vi "Farming Robot V1.vi"() -> ()   [LabVIEW 2021]
uses:
  <vilib>/myRIO/Express VI/Onboard Devices/LED/LED Express VI.xnode
  <vilib>/myRIO/Instrument Drivers/Onboard IO/DIO/vis/Write.vi
  <vilib>/myRIO/Instrument Drivers/Onboard IO/DIO/DIO.lvlib
  <vilib>/myRIO/Common/Instrument Driver Framework/myRIO v1.0/DIO/typedefs/DIO Channels Enum.ctl
  <vilib>/myRIO/Common/Instrument Driver Framework/myRIO v1.0/DIO/typedefs/DIO Channels List.ctl
  <vilib>/myRIO/Common/Instrument Driver Framework/Utilities/typedefs/Generic FPGA Reference.ctl
  <vilib>/myRIO/Common/Instrument Driver Framework/Utilities/typedefs/myRIO v1.0 Reference.ctl
  <vilib>/myRIO/Common/Instrument Driver Framework/Utilities/typedefs/Hardware Version Enum.ctl
  <vilib>/myRIO/Common/Instrument Driver Framework/Utilities/typedefs/myRIO Generic Hardware Reference.ctl
  <vilib>/myRIO/Instrument Drivers/Onboard IO/DIO/typedefs/DIO Reference.ctl
  <vilib>/myRIO/Instrument Drivers/Onboard IO/DIO/vis/myRIO DIO Open.xnode
  <vilib>/myRIO/Common/Instrument Driver Framework/Utilities/vis/Is FPGA Ref Available.vi
  <vilib>/myRIO/Common/Instrument Driver Framework/myRIO v1.0/DIO/vis/myRIO v1.1 Open DIO.vi
  <vilib>/userDefined/High Color/nirio_resource_hc.ctl
  <vilib>/myRIO/Express VI/Onboard IO/DO/DO Express VI.xnode
  <vilib>/myRIO/Express VI/Onboard IO/PWM/PWM Express VI.xnode
  <vilib>/myRIO/Instrument Drivers/Onboard IO/PWM/vis/Set Duty Cycle and Frequency.vi
  <vilib>/myRIO/Instrument Drivers/Onboard IO/PWM/PWM.lvlib
  <vilib>/myRIO/Instrument Drivers/Onboard IO/PWM/typedefs/PWM Configuration.ctl
  <vilib>/myRIO/Common/Instrument Driver Framework/myRIO v1.0/PWM/typedefs/PWM Channels Enum.ctl
  <vilib>/myRIO/Instrument Drivers/Onboard IO/PWM/typedefs/PWM Reference.ctl
  <vilib>/myRIO/Instrument Drivers/Onboard IO/PWM/vis/myRIO PWM Open.xnode
  <vilib>/myRIO/Common/Instrument Driver Framework/myRIO v1.0/PWM/vis/myRIO v1.1 Open PWM.vi
  <vilib>/Analysis/NI_AALPro.lvlib
  <vilib>/myRIO/Express VI/Onboard Devices/Accelerometer/Accelerometer Express VI.xnode
  <vilib>/myRIO/Instrument Drivers/Onboard Devices/Accelerometer/vis/Read.vi
  <vilib>/myRIO/Instrument Drivers/Onboard Devices/Accelerometer/Accelerometer.lvlib
  <vilib>/myRIO/Common/Instrument Driver Framework/myRIO v1.0/Accelerometer/typedefs/Accelerometer Channels Enum.ctl
  <vilib>/myRIO/Common/Instrument Driver Framework/myRIO v1.0/Accelerometer/typedefs/Accelerometer Channels List.ctl
  <vilib>/myRIO/Instrument Drivers/Onboard Devices/Accelerometer/typedefs/Accelerometer Reference.ctl
  <vilib>/myRIO/Instrument Drivers/Onboard Devices/Accelerometer/vis/myRIO Accelerometer Open.xnode
  <vilib>/myRIO/Common/Instrument Driver Framework/myRIO v1.0/Accelerometer/vis/myRIO v1.1 Open Accelerometer.vi
panel:
  in  "servo 1":dbl(slide) scale=0.0..180.0
  out "pulse width 1":dbl
  out "Angle 1":dbl
  in  "Duty Cycle":dbl(slide)=0.5 scale=0.0..1.0
  in  "Input 4":bool
  in  "Input 3":bool
  in  "Input 2":bool
  in  "Input 1":bool
  in  "Start Farming":bool
  out "Watering":bool
  out "Seeding\nUp":bool
  out "Seeding\nDown":bool
  out "Switching\nMode":bool
  out "Drill Up":bool
  out "Drill Down":bool
  out "Intialize":bool
  out "Message":string
  in  "stop":bool
  out "States":T1(ring)
  # "Motors"
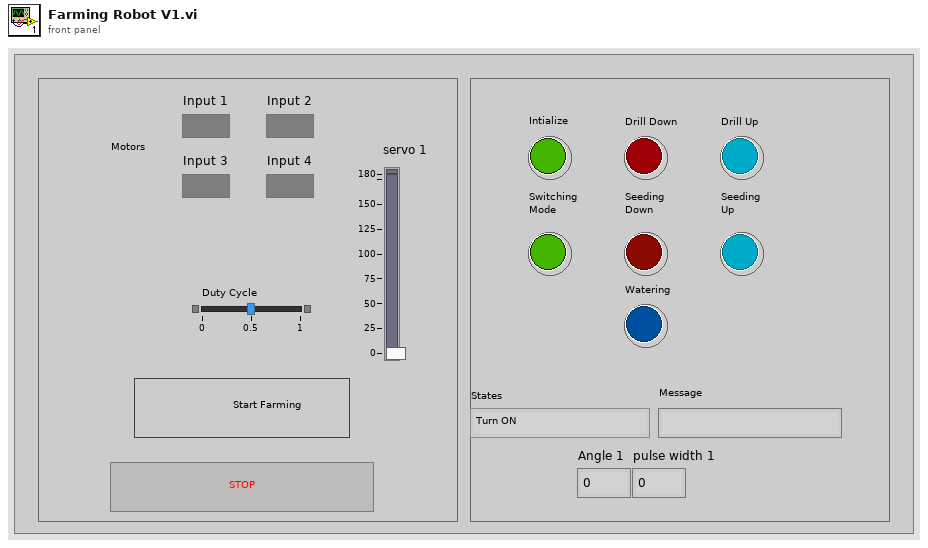
[diagram p1: front panel]
types:
  T1 = enum16{"Turn ON", "IDLE", "Start Farming", "Drive", "Seeding", "Watering", "Filling", "Fell off", "Stop", "Drill"}
  T2 = enum16{"Turn ON", "IDLE", "Start Farming", "Drive", "Seeding", "Watering", "Filling", "Fell off", "Stop"}
  T3 = typedef "DIO.lvlib/DIO Reference.ctl" = cluster{"myRIO Reference":T4, "DIO Channels List":T8}
  T4 = typedef "myRIO Generic Hardware Reference.ctl" = cluster{"myRIO Model":T5, "myRIO Hardware Reference":T6}
  T5 = typedef "Hardware Version Enum.ctl" = enum16{"Unknown", "myRIO-1900", "myRIO-1950", "roboRIO", "NI ELVIS RIO CM", "ELVIS III"}
  T6 = typedef "myRIO v1.0 Reference.ctl" = cluster{"Generic FPGA Reference":T7, "Allow multiple opens":bool}
  T7 = typedef "Generic FPGA Reference.ctl" = refnum<k20>
  T8 = typedef "DIO Channels List.ctl" = T9[]
  T9 = typedef "DIO Channels Enum.ctl" = enum16{"Not Connected", "C/DIO0", "C/DIO1", "C/DIO2", "C/DIO3", "C/DIO4", "C/DIO5", "C/DIO6", "C/DIO7", "A/DIO0", "A/DIO1", "A/DIO2", "A/DIO3", "A/DIO4", "A/DIO5", "A/DIO6", "A/DIO7", "A/DIO8", "A/DIO9", "A/DIO10", "A/DIO11", "A/DIO12", "A/DIO13", "A/DIO14", "A/DIO15", "A/DIO16", "A/DIO17", "A/DIO18", "A/DIO19", "B/DIO0", "B/DIO1", "B/DIO2", "B/DIO3", "B/DIO4", "B/DIO5", "B/DIO6", "B/DIO7", "B/DIO8", "B/DIO9", "B/DIO10", "B/DIO11", "B/DIO12", "B/DIO13", "B/DIO14", "B/DIO15", "B/DIO16", "B/DIO17", "B/DIO18", "B/DIO19", "LED0", "LED1", "LED2", "LED3", "Button0", "DIO/DIO0", "DIO/DIO1", "DIO/DIO2", "DIO/DIO3", "DIO/DIO4", "DIO/DIO5", "DIO/DIO6", "DIO/DIO7", "DIO/DIO8", "DIO/DIO9", "SPI/CS0", "SPI/CS1", "SPI/CS2", "SPI/CS3", "LED RADIO (Green)", "LED RADIO (Red)", "LED COMM (Green)", "LED COMM (Red)", "LED MODE (Green)", "LED MODE (Red)"}
  T10 = typedef "nirio_resource_hc.ctl" = tag
  T11 = typedef "Accelerometer.lvlib/Accelerometer Reference.ctl" = cluster{"myRIO Reference":T4, "Accelerometer Channels List":T12, "LSB Weight":dbl}
  T12 = typedef "Accelerometer Channels List.ctl" = T13[]
  T13 = typedef "Accelerometer Channels Enum.ctl" = enum16{"Not Connected", "X-Axis", "Y-Axis", "Z-Axis"}
  T14 = typedef "PWM.lvlib/PWM Reference.ctl" = cluster{"myRIO Reference":T4, "PWM Channels Enum":T15, "PWM Configuration":T16}
  T15 = typedef "PWM Channels Enum.ctl" = enum16{"Not Connected", "C/PWM0", "C/PWM1", "A/PWM0", "A/PWM1", "A/PWM2", "A/PWM3", "A/PWM4", "A/PWM5", "A/PWM6", "A/PWM7", "A/PWM8", "A/PWM9", "A/PWM10", "A/PWM11", "A/PWM12", "A/PWM13", "A/PWM14", "A/PWM15", "A/PWM16", "A/PWM17", "A/PWM18", "A/PWM19", "B/PWM0", "B/PWM1", "B/PWM2", "B/PWM3", "B/PWM4", "B/PWM5", "B/PWM6", "B/PWM7", "B/PWM8", "B/PWM9", "B/PWM10", "B/PWM11", "B/PWM12", "B/PWM13", "B/PWM14", "B/PWM15", "B/PWM16", "B/PWM17", "B/PWM18", "B/PWM19", "PWM/PWM0", "PWM/PWM1", "PWM/PWM2", "PWM/PWM3", "PWM/PWM4", "PWM/PWM5", "PWM/PWM6", "PWM/PWM7", "PWM/PWM8", "PWM/PWM9"}
  T16 = typedef "PWM.lvlib/PWM Configuration.ctl" = cluster{"Frequency":dbl, "Duty Cycle":dbl}
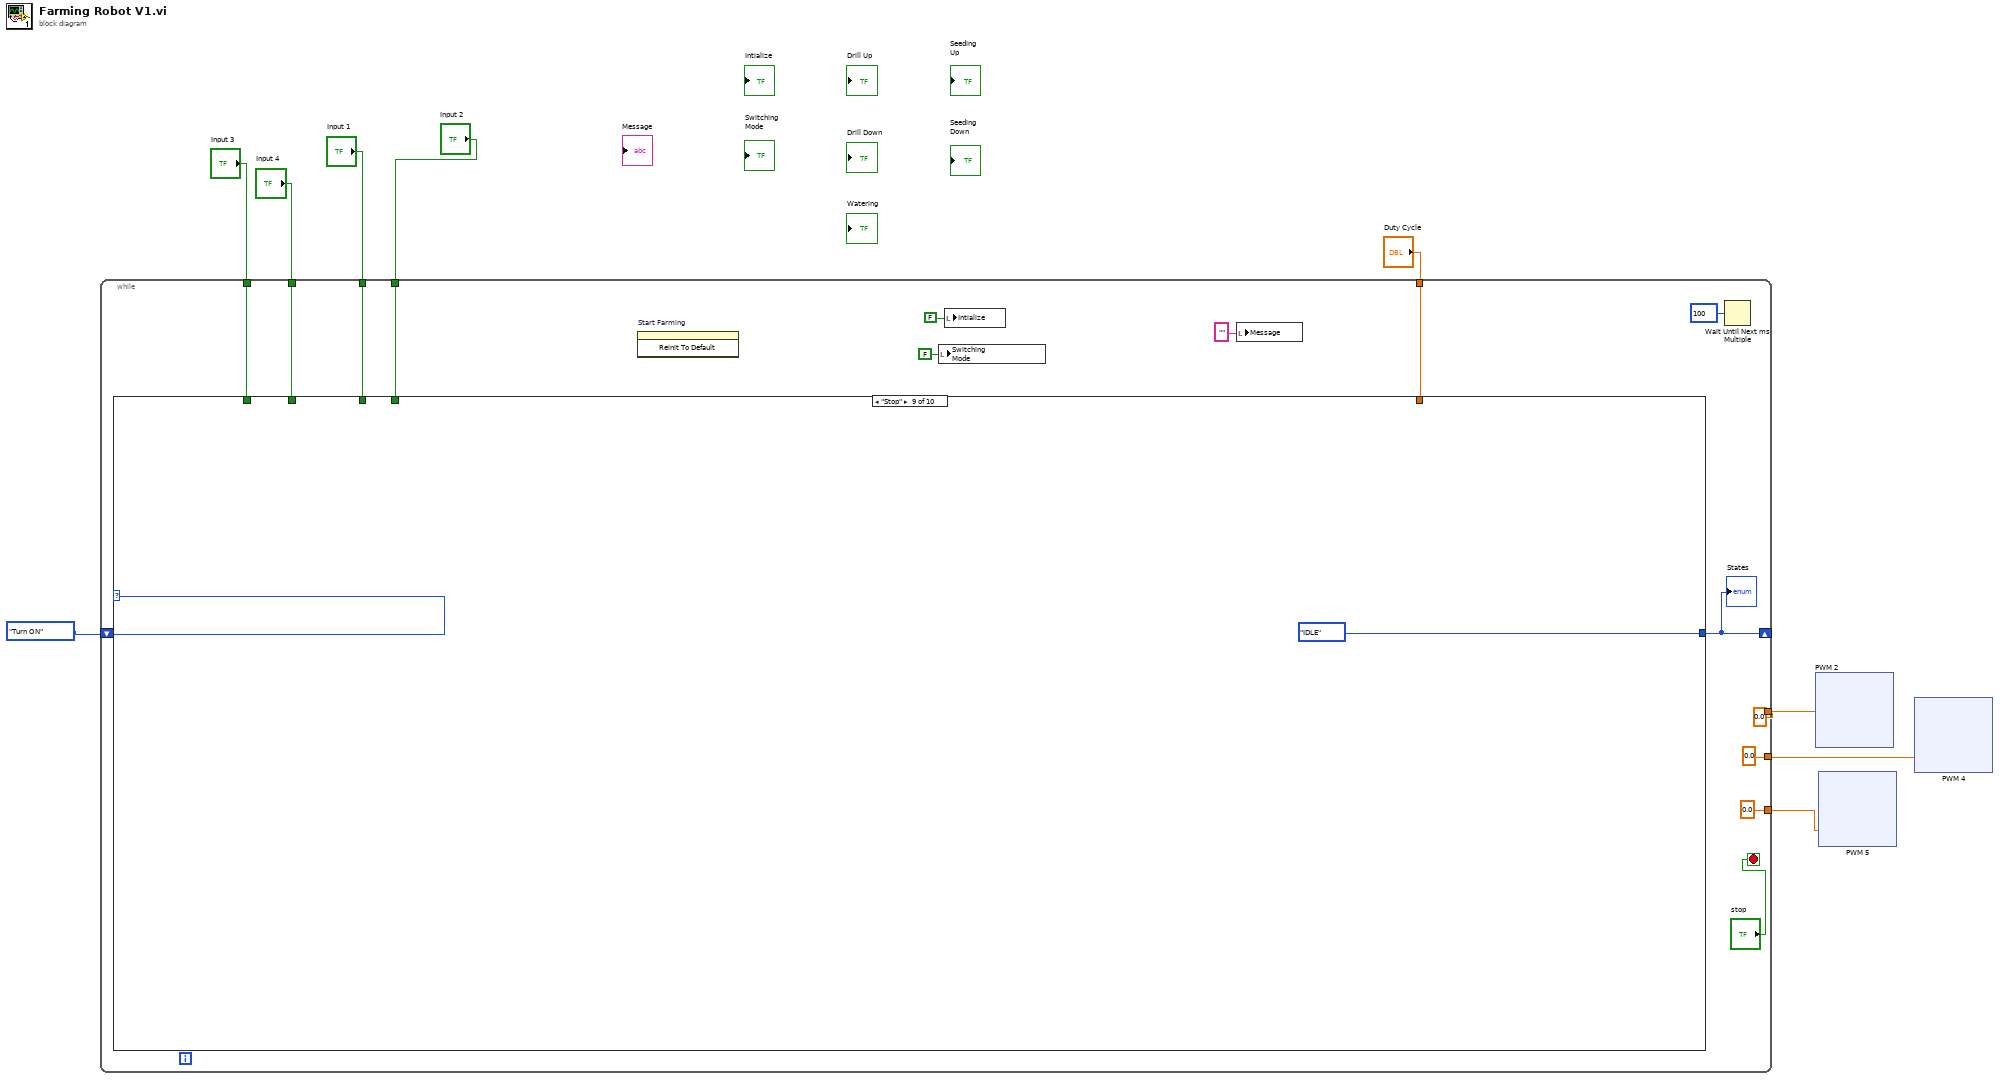
[diagram p0: block diagram]
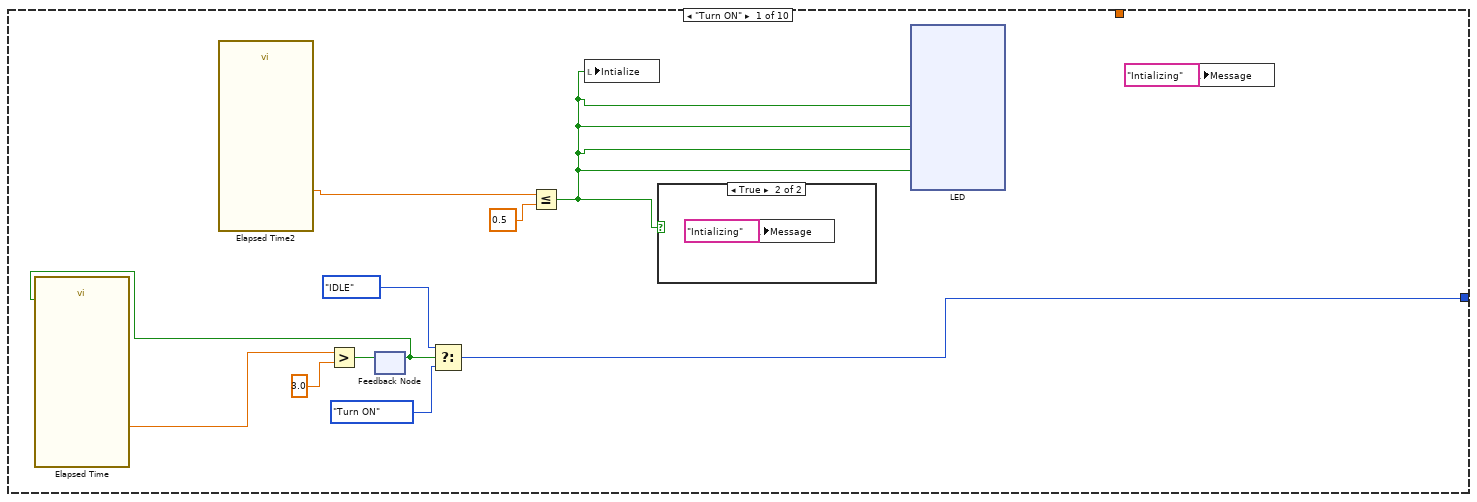
[diagram p2: hidden frame]
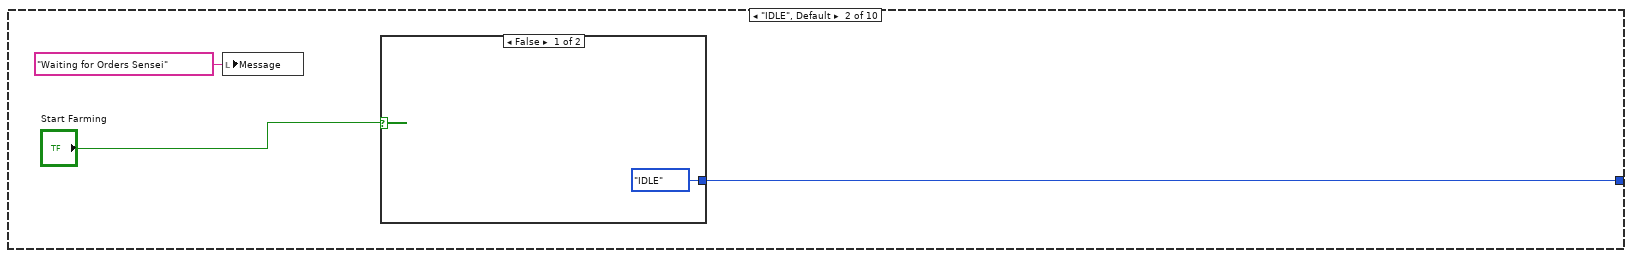
[diagram p4: hidden frame]
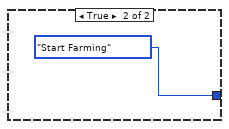
[diagram p5: hidden frame]
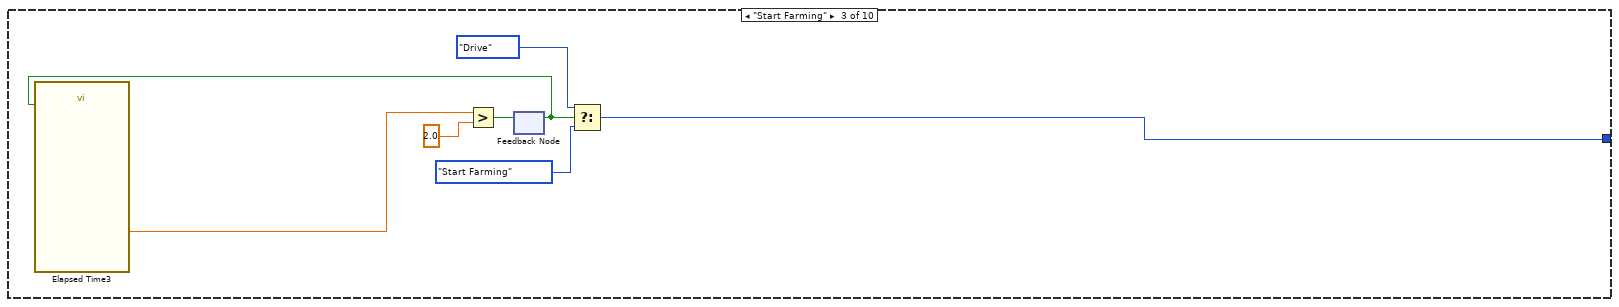
[diagram p6: hidden frame]
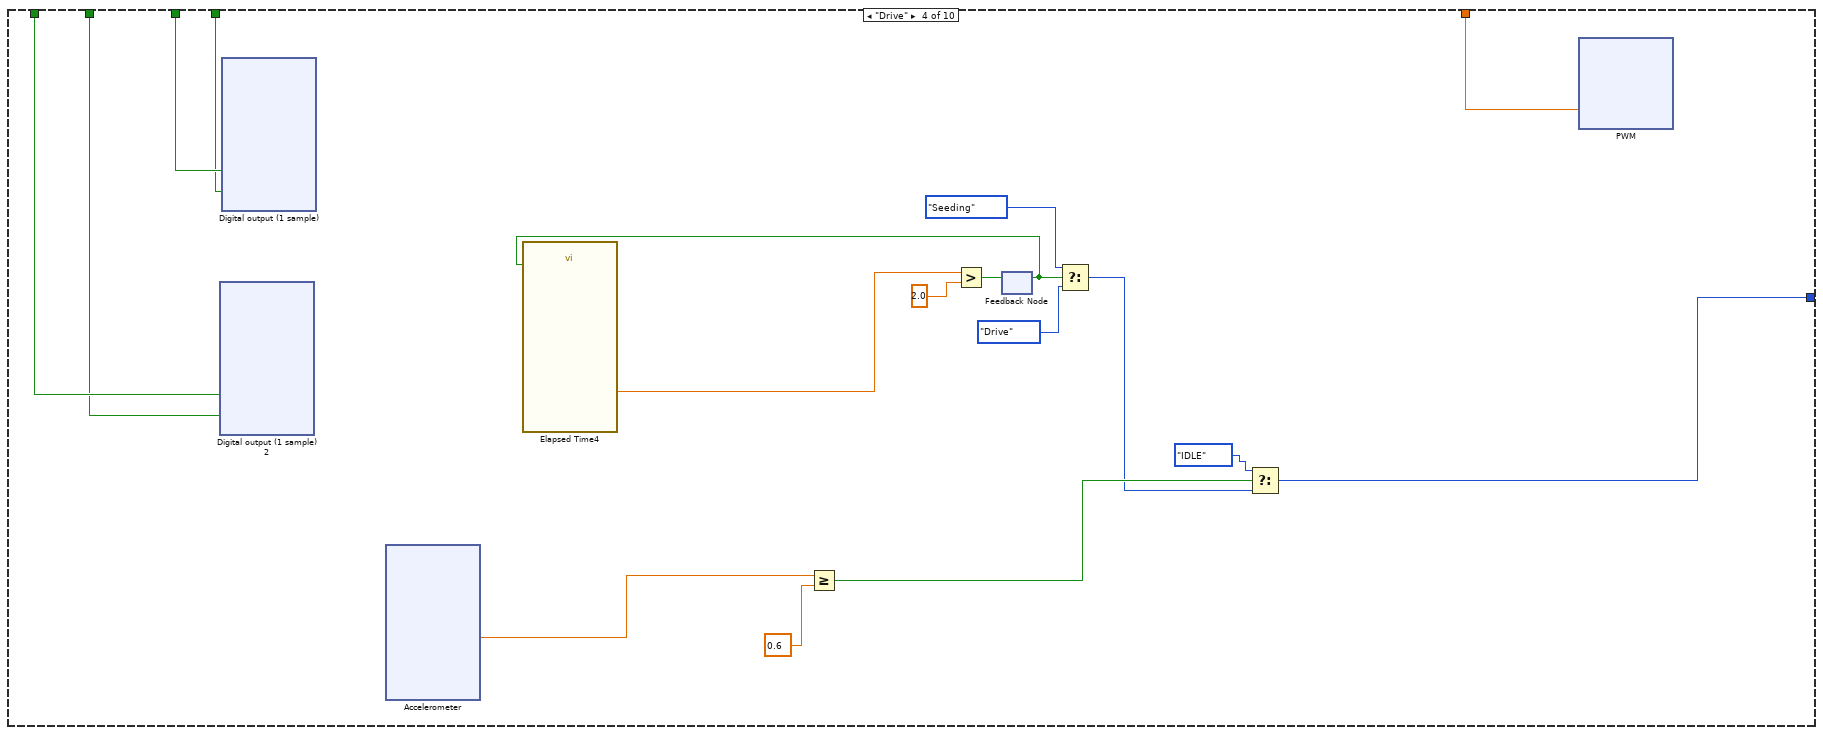
[diagram p7: hidden frame]
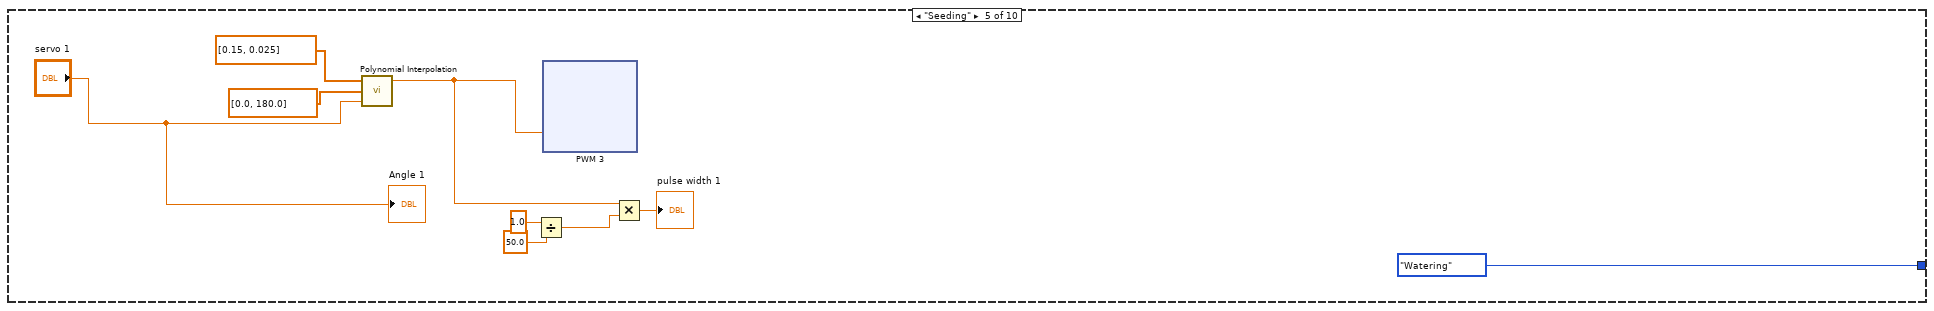
[diagram p8: hidden frame]
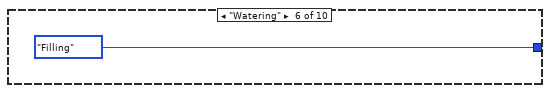
[diagram p9: hidden frame]
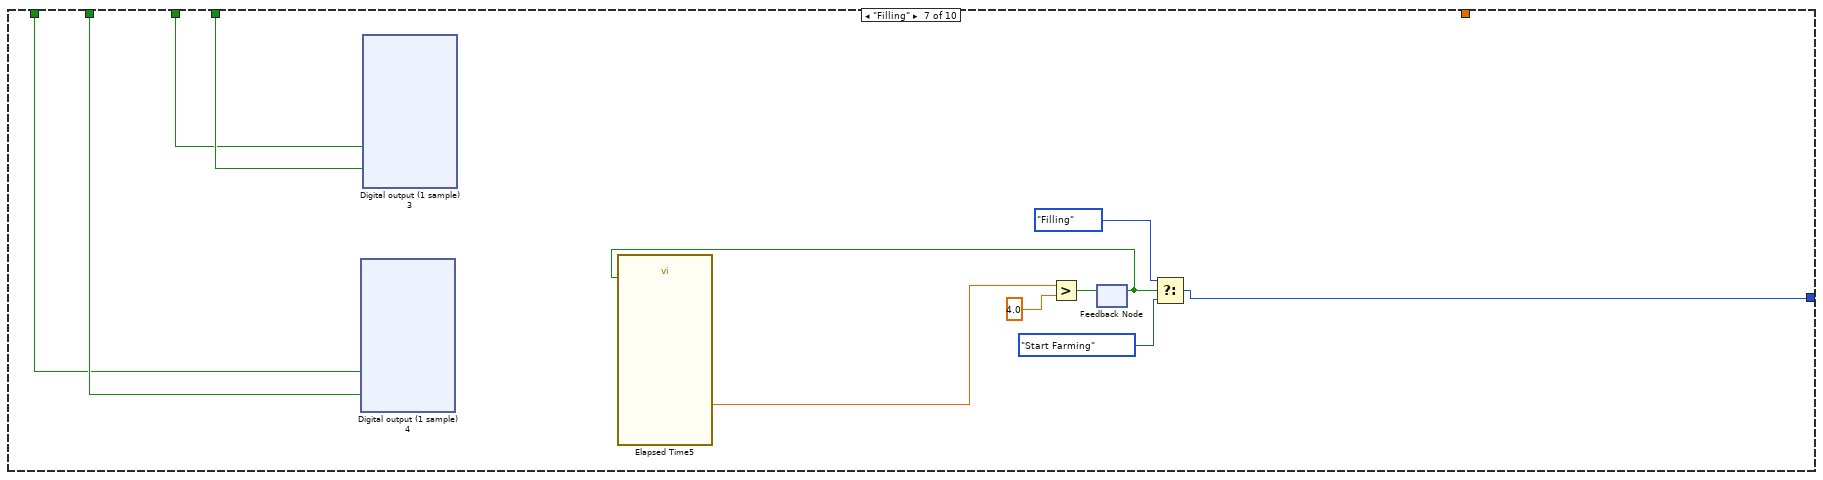
[diagram p10: hidden frame]
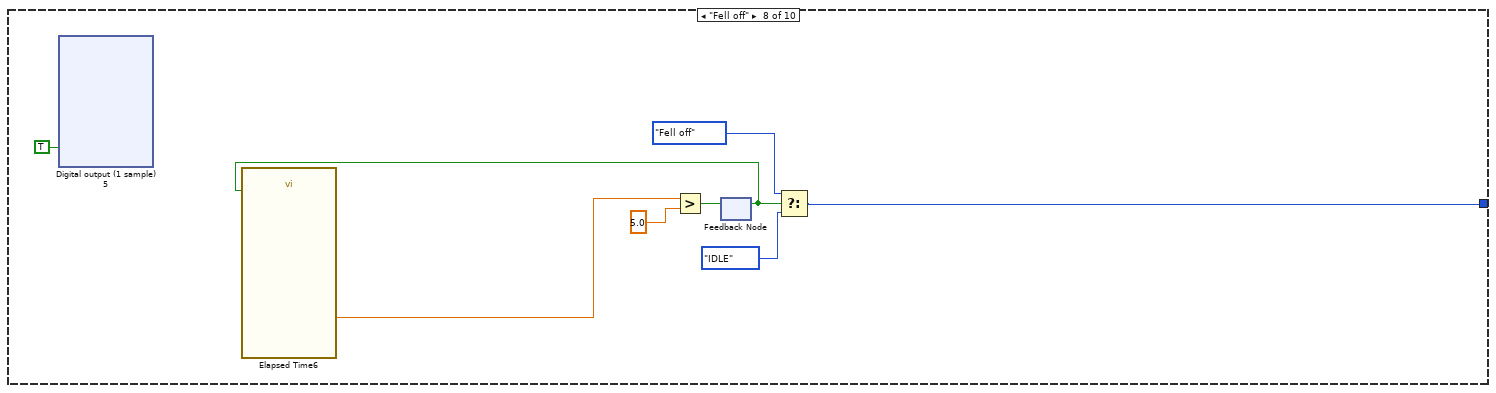
[diagram p11: hidden frame]
diagram:
  n1 = while {
    shift-right: [w22] -> _
    shift-left: T1."Turn ON" ("States") -> [w24]
    tunnel: [0.0 ("Duty Cycle")] -> w9
    tunnel: "Input 1" -> [w16]
    tunnel: "Input 2" -> [w15]
    tunnel: "Input 3" -> [w14]
    tunnel: "Input 4" -> [w13]
    tunnel: [0.0 ("Duty Cycle")] -> w4
    tunnel: [0.0 ("Duty Cycle")] -> w3
    tunnel: "Duty Cycle" -> [w10]
    stop <- "stop" stop-if-true
    n2 = case shown="\"Stop\"" w24 {
      tunnel: [w31 w77 w80 w90 T2."Watering" ("States") T2."Filling" ("States") w295 w378 T2."IDLE" ("States") _] -> w22
      tunnel: w16 -> [_ _ _ w103 _ _ w304 _ _ _]
      tunnel: w15 -> [_ _ _ w102 _ _ w305 _ _ _]
      tunnel: w14 -> [_ _ _ w101 _ _ w302 _ _ _]
      tunnel: w13 -> [_ _ _ w100 _ _ w303 _ _ _]
      tunnel: w10 -> [_ _ _ w87 _ _ _ _ _ _]
      frame "Turn ON" {
        n3 = call "Elapsed Time2"() -> ("Elapsed Time (s)"=w28:dbl)  [unwired: 12 in, 7 out]
        n4 = feedback #1() -> (w29:bool)  [unwired: 1 in]
        n5 = call "Elapsed Time"("Reset"=w29) -> ("Elapsed Time (s)"=w35:dbl)  [unwired: 11 in, 7 out]
        n6 = Greater?(x=w35, y=3.0) -> (0:w30:bool)
        n7 = feedback-in #1(w30) -> ()
        n8 = Select(t=T2."IDLE" ("States"), s=w29, f=T2."Turn ON" ("States")) -> (s? t:f=w31:T2)
        n9 = Less Or Equal?(x=w28, y=0.5) -> (x <= y?=w25:bool)
        n10 = local write "Intialize"(w25) -> ()
        n11 = case shown="True" w25 {
          frame False {
          }
          frame True {
            n12 = local write "Message"("Intializing" ("msg")) -> ()
          }
        }
        n13 = xnode "LED"("LED0"=w25, "LED1"=w25, "LED2"=w25, "LED3"=w25) -> ()  [unwired: 1 in, 1 out]
        n14 = local write "Message"("Intializing" ("msg")) -> ()
      }
      frame "IDLE", Default {
        n15 = local write "Message"("Waiting for Orders Sensei" ("Message")) -> ()
        n16 = case shown="False" "Start Farming" {
          tunnel: [T2."IDLE" ("States") T2."Start Farming" ("States")] -> w77
          frame False {
          }
          frame True {
          }
        }
      }
      frame "Start Farming" {
        n17 = feedback #2() -> (w81:bool)  [unwired: 1 in]
        n18 = call "Elapsed Time3"("Reset"=w81) -> ("Elapsed Time (s)"=w86:dbl)  [unwired: 11 in, 7 out]
        n19 = Greater?(x=w86, y=2.0) -> (0:w82:bool)
        n20 = feedback-in #2(w82) -> ()
        n21 = Select(t=T2."Drive" ("States"), s=w81, f=T2."Start Farming" ("States")) -> (s? t:f=w80:T2)
      }
      frame "Drive" {
        n22 = xnode "Digital output (1 sample) 2"("A/DIO2 (Pin 15)"=w101, "A/DIO3 (Pin 17)"=w100) -> ()  [unwired: 1 in, 1 out]
        n23 = xnode "Digital output (1 sample)"("A/DIO0 (Pin 11)"=w103, "A/DIO1 (Pin 13)"=w102) -> ()  [unwired: 1 in, 1 out]
        n24 = xnode "Accelerometer"() -> ("X-Axis"=w92:dbl)  [unwired: 1 in, 3 out]
        n25 = Greater Or Equal?(x=w92, y=0.6) -> (x >= y?=w91:bool)
        n26 = feedback #3() -> (w94:bool)  [unwired: 1 in]
        n27 = call "Elapsed Time4"("Reset"=w94) -> ("Elapsed Time (s)"=w99:dbl)  [unwired: 11 in, 7 out]
        n28 = Greater?(x=w99, y=2.0) -> (0:w95:bool)
        n29 = feedback-in #3(w95) -> ()
        n30 = Select(t=T2."Seeding" ("States"), s=w94, f=T2."Drive" ("States")) -> (s? t:f=w89:T2)
        n31 = Select(t=T2."IDLE" ("States"), s=w91, f=w89) -> (s? t:f=w90:T2)
        n32 = xnode "PWM"("Duty Cycle"=w87) -> ()  [unwired: 1 in, 1 out]
      }
      frame "Seeding" {
        n33 = call <vilib>:"Polynomial Interpolation.vi"("x value"="servo 1", "X"=dbl[] [0.0, 180.0], "Y"=dbl[] [0.15, 0.025]) -> ("interpolation value"=w252:dbl)  [unwired: 2 out]
        n34 = Divide(x=1.0, y=50.0) -> (x/y=w253:dbl)
        n35 = xnode "PWM 3"("Duty Cycle"=w252) -> ()  [unwired: 1 in, 1 out]
        n36 = Multiply(x=w252, y=w253) -> (x*y=→"pulse width 1":dbl)
        "Angle 1" <- "servo 1"
      }
      frame "Watering" {
      }
      frame "Filling" {
        n37 = xnode "Digital output (1 sample) 4"("A/DIO2 (Pin 15)"=w302, "A/DIO3 (Pin 17)"=w303) -> ()  [unwired: 1 in, 1 out]
        n38 = xnode "Digital output (1 sample) 3"("A/DIO0 (Pin 11)"=w304, "A/DIO1 (Pin 13)"=w305) -> ()  [unwired: 1 in, 1 out]
        n39 = feedback #4() -> (w296:bool)  [unwired: 1 in]
        n40 = call "Elapsed Time5"("Reset"=w296) -> ("Elapsed Time (s)"=w301:dbl)  [unwired: 11 in, 7 out]
        n41 = Greater?(x=w301, y=4.0) -> (0:w297:bool)
        n42 = feedback-in #4(w297) -> ()
        n43 = Select(t=T2."Filling" ("States"), s=w296, f=T2."Start Farming" ("States")) -> (s? t:f=w295:T2)
      }
      frame "Fell off" {
        n44 = xnode "Digital output (1 sample) 5"("A/DIO4 (Pin 19)"=TRUE) -> ()  [unwired: 1 in, 1 out]
        n45 = feedback #5() -> (w379:bool)  [unwired: 1 in]
        n46 = call "Elapsed Time6"("Reset"=w379) -> ("Elapsed Time (s)"=w384:dbl)  [unwired: 11 in, 7 out]
        n47 = Greater?(x=w384, y=5.0) -> (0:w380:bool)
        n48 = feedback-in #5(w380) -> ()
        n49 = Select(t=T2."Fell off" ("States"), s=w379, f=T2."IDLE" ("States")) -> (s? t:f=w378:T2)
      }
      frame "Stop" {
      }
      frame "Drill" {
      }
    }
    "States" <- w22
    n50 = invoke on="Start Farming" class="Bool" method="Reinit To Default"() -> ()  [unwired: 3 in, 3 out]
    n51 = local write "Switching\nMode"(FALSE ("Switching\nMode")) -> ()
    n52 = local write "Intialize"(FALSE ("Intialize")) -> ()
    n53 = local write "Message"("" ("Message")) -> ()
    n54 = Wait Until Next ms Multiple(millisecond multiple=u32 100) -> ()  [unwired: 1 out]
  }
  n55 = xnode "PWM 2"("Duty Cycle"=w9) -> ()  [unwired: 1 in, 1 out]
  n56 = xnode "PWM 5"("Duty Cycle"=w3) -> ()  [unwired: 1 in, 1 out]
  n57 = xnode "PWM 4"("Duty Cycle"=w4) -> ()  [unwired: 1 in, 1 out]
